vi "DHTxx Temp-Humidity Sensor.vi"() -> ()   [LabVIEW 2014]
doc: "This example shows how to read temp data from DHTxx sensor."
uses:
  QwaveSys_Interface/QwaveSys_Interface.lvlib
  PWS_ESP8266/PWS_ESP8266.lvlib
panel:
  in  "DHTxx":u8(ring)=15 items=["SPI#1/SS,(5)"=5, "SPI#2/MOSI,(13)"=13, "SPI#3/MISO,(12)"=12, "SPI#4/SCLK,(14)"=14, "UART#1/CS,(15)"=15, "UART#2/TXD,(1)"=1, "UART#3/RXD,(3)"=3, "UART#4/LED,(16)"=16, "FPROM_Btn,(0)"=0, "SDCard_CS,(4)"=4, "I2C-SDA/TXD1,(2)"=2, "ADC0,(17)"=17]
  # "Overview: Demonstrates how to read  DHTxx sensor connected to digital pin.\nRequirements: LabVIEW Full Development System,Arduino Compatible Compiler for LabVIEW,Programmable Wireless Stamp (PWS) Library.\nInstructions:\n1. Wire a temperature sensor DHTxx (This example using DHT22) as specified below where the data pin is wired to the specified Digital Pin (GPIO15) below.\n2.  If this example has been loaded from the Arduino Compatible Compiler for LabVIEW, simply select Compile and Download.  Otherwise, open Tools>Arduino Compatible Compiler for LabVIEW in LabVIEW, then select File>Load VI, and select this VI and then Compile and Download.\n3. Open \"Serial Monitor\" by select \"Tools>Serial Monitor\" and select baud rate to 9600.\n4. Observe the logged data being print out on serial port monitor."
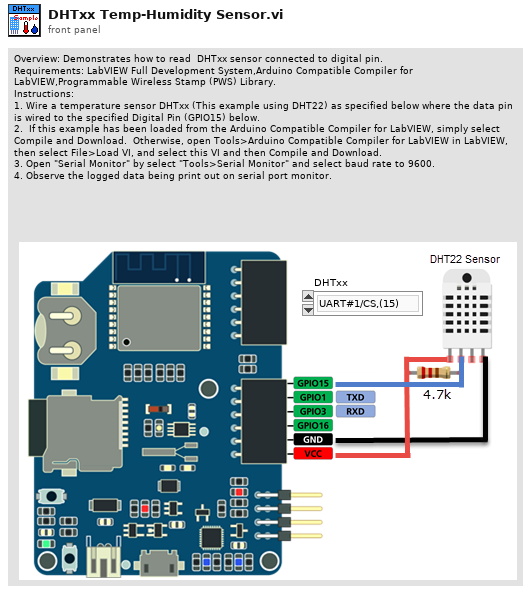
[diagram p1: front panel]
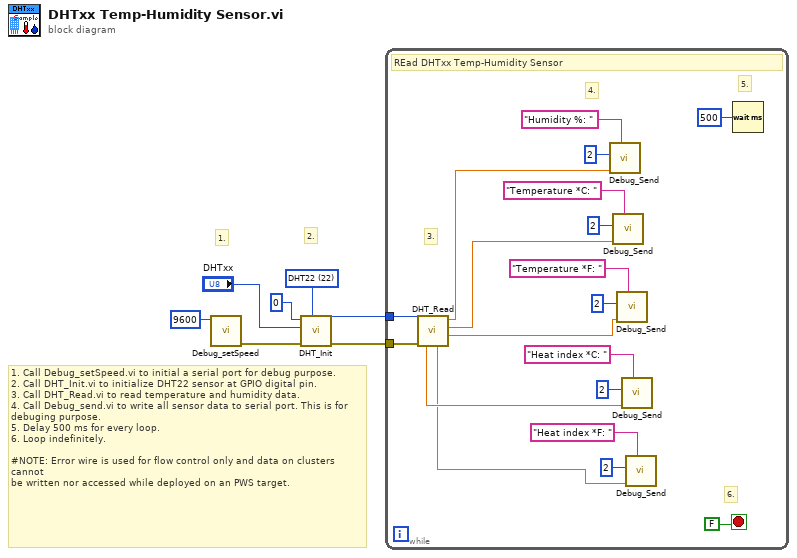
[diagram p0: block diagram]
diagram:
  w4 = u16 22 items=["DHT11"=11, "DHT21"=21, "DHT22"=22] ("Type")
  # "1. Call Debug_setSpeed.vi to initial a serial port for debug purpose.\n2. Call DHT_Init.vi to initialize DHT22 sensor at GPIO digital pin. \n3. Call DHT_Read.vi to read temperature and humidity data.\n4. Call Debug_send.vi to write all sensor data to serial port. This is for debuging purpose.\n5. Delay 500 ms for every loop.\n6. Loop indefinitely.\n\n#NOTE: Error wire is used for flow control only and data on clusters cannot\nbe written nor accessed while deployed on an PWS target."
  # "2."
  # "1."
  n1 = call "Debug_setSpeed.vi"("Speed"=u32 9600) -> ("error out"=w2:errorcluster)  [unwired: 10 in]
  n2 = call "DHT_Init.vi"("Type"=w4, "error in (no error)"=w2, "PIN"="DHTxx", "Interface (0-4)"=u8 0) -> ("error out"=w6:errorcluster, "Instance"=w5:u8)  [unwired: 6 in]
  n3 = while {
    tunnel: w6 -> [w26]
    tunnel: w5 -> [w22]
    stop <- FALSE stop-if-true
    # "6."
    # "5."
    # "4."
    # "3."
    # "REad DHTxx Temp-Humidity Sensor"
    n4 = call "DHT_Read.vi"("Instance"=w22, "error in (no error)"=w26) -> ("Fahrenheit"=w10:dbl, "Celsius"=w11:dbl, "Humidity"=w12:dbl, "Heat Index (Fahrenheit)"=w8:dbl, "Heat Index (Celsius)"=w9:dbl)  [unwired: 4 in, 1 out]
    n5 = call "Debug_Send.vi"("Name"="Humidity %: ", "DATA"=w12, "Option"=2) -> ()  [unwired: 9 in]
    n6 = call "Debug_Send.vi"("Name"="Temperature *C: ", "DATA"=w11, "Option"=2) -> ()  [unwired: 9 in]
    n7 = call "Debug_Send.vi"("Name"="Temperature *F: ", "DATA"=w10, "Option"=2) -> ()  [unwired: 9 in]
    n8 = call "Debug_Send.vi"("Name"="Heat index *C: ", "DATA"=w9, "Option"=2) -> ()  [unwired: 9 in]
    n9 = call "Debug_Send.vi"("Name"="Heat index *F: ", "DATA"=w8, "Option"=2) -> ()  [unwired: 9 in]
    n10 = Wait (ms)(milliseconds to wait=u32 500) -> ()  [unwired: 1 out]
  }
